vi "Read Q0 params.vi"(8 "error in (no error)":errorcluster, 11 "Scope5761 in":refnum<class "Scope5782_six_channel.lvclass">) -> (0 "error out":errorcluster, 2 "Q0 params":T1, 3 "Scope5761out":refnum<class "Scope5782_six_channel.lvclass">)   [LabVIEW 2018, in "Scope5782_six_channel.lvclass"]
uses:
  Scope5782_six_channel.lvclass
  Q0 params.ctl
  Scope5782_six_channel.lvclass/Scope5782_six_channel.ctl
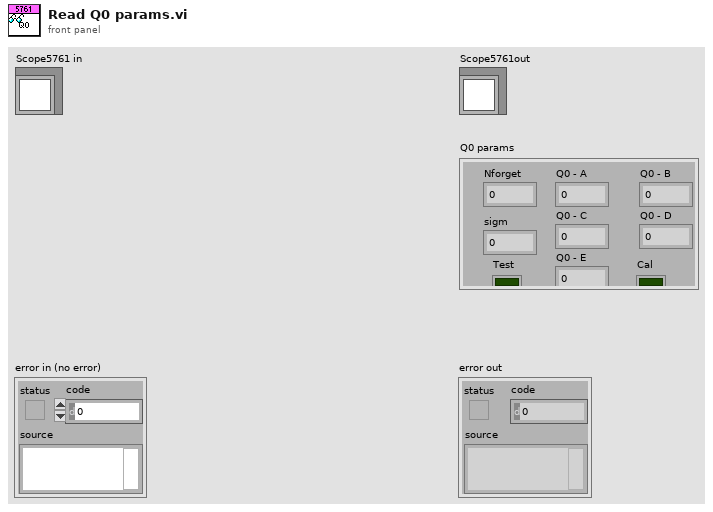
[diagram p1: front panel]
types:
  T1 = typedef "Scope5782_six_channel.lvclass/Q0 params.ctl" = cluster{"Nforget":i32, "sigm":dbl, "Q0 - A":dbl, "Q0 - B":dbl, "Q0 - C":dbl, "Q0 - D":dbl, "Q0 - E":dbl, "Test":bool, "Cal":bool}
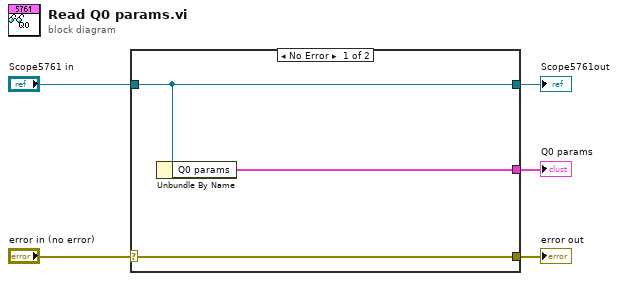
[diagram p0: block diagram]
diagram:
  n1 = case shown="No Error" "error in (no error)" {
    selector: "error in (no error)" -> [w8 w9]
    tunnel: [w8 w9] -> w4
    tunnel: [w7 w10] -> w2
    tunnel: "Scope5761 in" -> [w7 w10]
    tunnel: [w6 _] -> w1
    frame No Error {
      n2 = Unbundle By Name(w7) -> ("Q0 params"=w6:T1)
    }
    frame Error {
    }
  }
  "error out" <- w4
  "Scope5761out" <- w2
  "Q0 params" <- w1
